vi "Refresh Step.vi"(6 "Skip Response? (F)":bool, 8 "error in (no error)":errorcluster, 10 "Step":refnum<class "Step.lvclass">, 11 "SequenceViewPanel in":refnum<class "SequenceViewPanel.lvclass">) -> (0 "error out":errorcluster, 3 "SequenceViewPanel out":refnum<class "SequenceViewPanel.lvclass">)   [LabVIEW 2020, in "TSnax UI.lvlib" / "SequenceViewPanel.lvclass"]
uses:
  SequenceViewPanel.lvclass
  SequenceViewPanel.lvclass/SequenceViewPanel.ctl
  cbcb8ed2-cbbd-406c-8d93-3c8802933451.vi
  TSnax/Step/Step.lvclass
  Error Response.ctl
  TSnax UI.lvlib
  Refresh Step Request.ctl
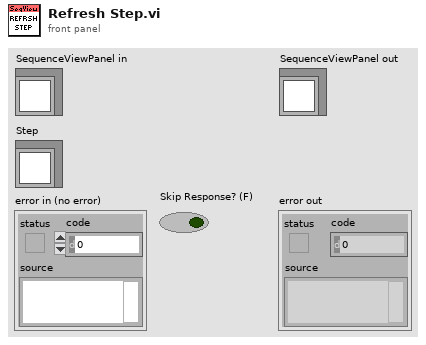
[diagram p1: front panel]
types:
  T1 = typedef "TSnax UI.lvlib/SequenceViewPanel.lvclass/Refresh Step Request.ctl" = cluster{"Step":refnum<class "Step.lvclass">, "Notifier":refnum<notifier>, "Auto-Release":bool}
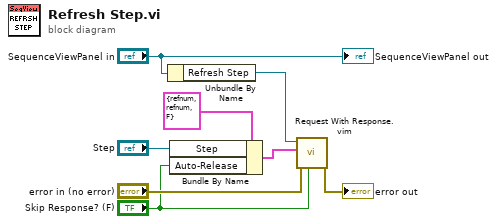
[diagram p0: block diagram]
diagram:
  n1 = Unbundle By Name("SequenceViewPanel in") -> ("Refresh Step"=w7:refnum<user-event>)
  n2 = Bundle By Name(cluster=T1 {"Step"=refnum, "Notifier"=refnum, "Auto-Release"=FALSE} ("Refresh Step Request"), "Step"="Step", "Auto-Release"="Skip Response? (F)") -> (w4:T1)
  n3 = call "Request With Response.vim"("Skip Response? (F)"="Skip Response? (F)", "error in (no error)"="error in (no error)", "Request Data"=w4, "Event"=w7) -> ("error out"=→"error out":errorcluster)  [unwired: 6 in, 1 out]
  "SequenceViewPanel out" <- "SequenceViewPanel in"
